vi "SATTPdll.vi"(8 "error in (no error)":errorcluster, 11 "SAT Inputs":T2={"t"=0.0, "p"=0.0, "z"=[0.0, 0.0, 0.0, 0.0, 0.0, 0.0, 0.0, 0.0, 0.0, 0.0, 0.0, 0.0, 0.0, 0.0, 0.0, 0.0, 0.0, 0.0, 0.0, 0.0], "kph"=0, "iGuess"=0} {"kph" items=["0 - Flash calculation (T and P known)", "1 - T and xliq known, P and xvap returned", "2 - T and xvap known, P and xliq returned", "3 - P and xliq known, T and xvap returned", "4 - P and xvap known, T and xliq returned"]}) -> (0 "error out":errorcluster, 3 "SAT Outputs":T1={"D"=nan, "e"=nan, "h"=nan, "p"=nan, "s"=nan, "t"=nan, "q"=nan, "Dl"=nan, "Dv"=nan, "x"=[nan, nan, 0.0, 0.0, 0.0, 0.0, 0.0, 0.0, 0.0, 0.0, 0.0, 0.0, 0.0, 0.0, 0.0, 0.0, 0.0, 0.0, 0.0, 0.0], "y"=[nan, nan, 0.0, 0.0, 0.0, 0.0, 0.0, 0.0, 0.0, 0.0, 0.0, 0.0, 0.0, 0.0, 0.0, 0.0, 0.0, 0.0, 0.0, 0.0], "nroot"=0, "k1"=0, "t1"=nan, "p1"=nan, "d1"=nan, "k2"=0, "t2"=nan, "p2"=nan, "d2"=nan, "k3"=0, "t3"=nan, "p3"=nan, "d3"=nan, "ierr"=0, "herr"="", "herr_length"=0})   [LabVIEW 2016]
doc: "subroutine SATTPdll(t, p, z, kph, iguess, d, dl, dv, x, y, q, ierr, herr, herr_length)\n\nCalculate saturation properties for bubble, dew, or 2-phase states with the use of analytical derivatives of the Helmholtz energy with respect to composition.\n\nINPUTS:\n t--temperature [K] (input or output)\n p--pressure [MPa] (input or output)\n z--composition [array of mol frac]\n kph--Phase flag: 0 - Flash calculation (T and P known)\n 1 - T and x known, P and y returned\n 2 - T and y known, P and x returned\n 3 - P and x known, T and y returned\n 4 - P and y known, T and x returned\n if this value is negative, the retrograde point will be returned\n iGuess--if set to 1, all inputs are used as initial guesses for the calculation\n\nOUTPUTS:\n D--overall molar density [mol/L]\n Dl--molar density [mol/L] of saturated liquid\n Dv--molar density [mol/L] of saturated vapor\n x--liquid phase composition [array of mol frac]\n y--vapor phase composition [array of mol frac]\n q--quality\n ierr--error flag: 0 = successful\n 1 = unsuccessful\n herr--error string (character*255 variable if ierr<>0)\n herr_length-- length of variable herr (default: 255)"
uses:
  Ctl/SAT_Outputs.ctl
  REFPROP.DLL
panel:
  # "REFPROP-SATTP_dll.vi"
  # "subroutine SATTPdll(t, p, z, kph, iguess, d, dl, dv, x, y, q, ierr, herr, herr_length)"
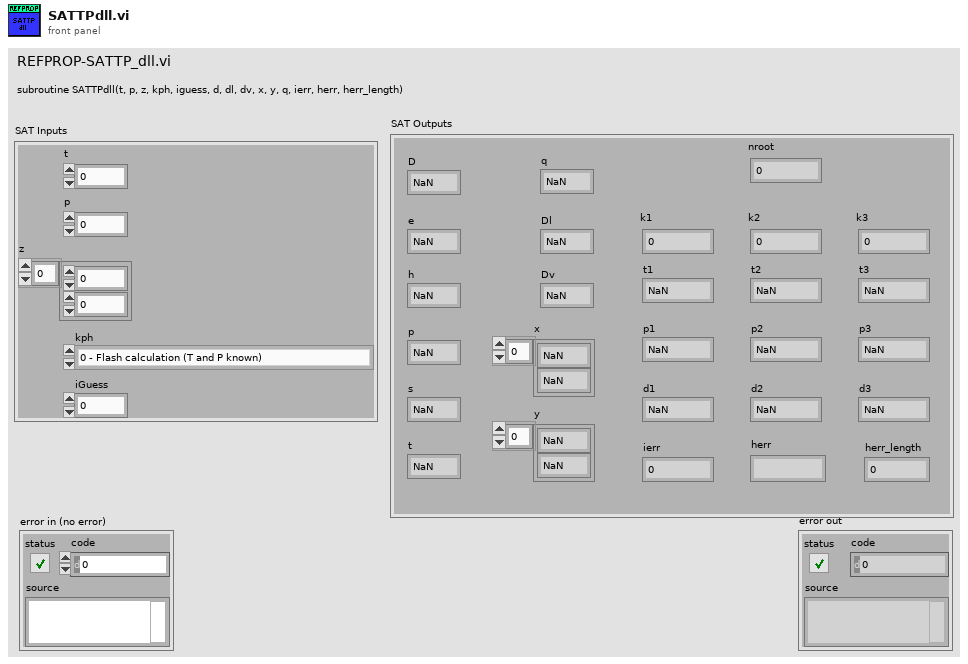
[diagram p1: front panel]
types:
  T1 = typedef "SAT_Outputs.ctl" = cluster{"D":dbl, "e":dbl, "h":dbl, "p":dbl, "s":dbl, "t":dbl, "q":dbl, "Dl":dbl, "Dv":dbl, "x":dbl[], "y":dbl[], "nroot":i32, "k1":i32, "t1":dbl, "p1":dbl, "d1":dbl, "k2":i32, "t2":dbl, "p2":dbl, "d2":dbl, "k3":i32, "t3":dbl, "p3":dbl, "d3":dbl, "ierr":i32, "herr":string, "herr_length":i32}
  T2 = cluster{"t":dbl, "p":dbl, "z":dbl[], "kph":u16, "iGuess":i32}
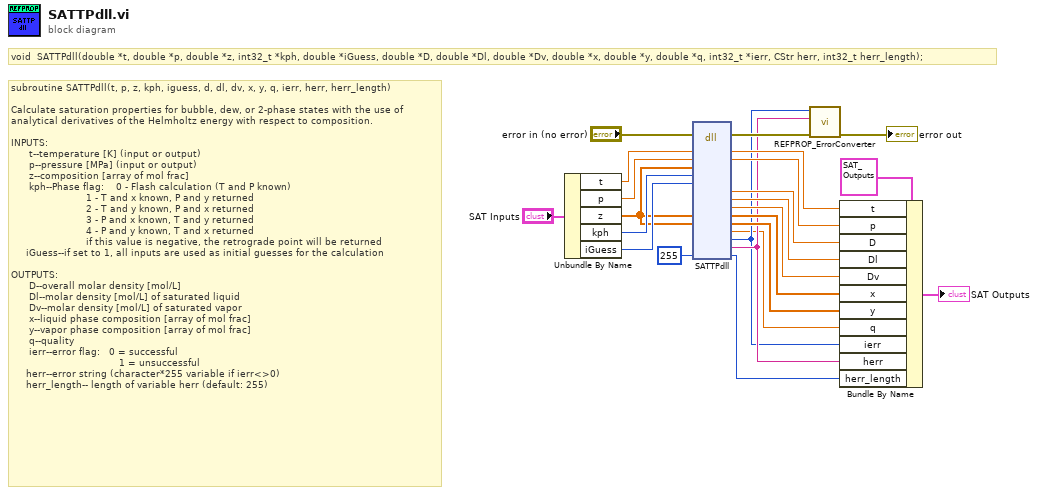
[diagram p0: block diagram]
diagram:
  # "void  SATTPdll(double *t, double *p, double *z, int32_t *kph, double *iGuess, double *D, double *Dl, double *Dv, double *x, double *y, double *q, int32_t *ierr, CStr herr, int32_t herr_length);"
  # "subroutine SATTPdll(t, p, z, kph, iguess, d, dl, dv, x, y, q, ierr, herr, herr_length)\n\nCalculate saturation properties for bubble, dew, or 2-phase states with the use of analytical derivatives of the Helmholtz energy with respect to composition.\n\nINPUTS:\n      t--temperature [K] (input or output)\n      p--pressure [MPa] (input or output)\n      z--composition [array of mol frac]\n      kph--Phase flag:    0 - Flash calculation (T and P known)\n                         1 - T and x known, P and y returned\n                         2 - T and y known, P and x returned\n                         3 - P and x known, T and y returned\n                         4 - P and y known, T and x returned\n                         if this value is negative, the retrograde point will be returned\n     iGuess--if set to 1, all inputs are used as initial guesses for the calculation\n\nOUTPUTS:\n      D--overall molar density [mol/L]\n      Dl--molar density [mol/L] of saturated liquid\n      Dv--molar density [mol/L] of saturated vapor\n      x--liquid phase composition [array of mol frac]\n      y--vapor phase composition [array of mol frac]\n      q--quality\n      ierr--error flag:   0 = successful\n                                    1 = unsuccessful\n     herr--error string (character*255 variable if ierr<>0)\n     herr_length-- length of variable herr (default: 255)"
  n1 = Unbundle By Name("SAT Inputs") -> ("t"=w21:dbl, "p"=w20:dbl, "z"=w14:dbl[], "kph"=w19:u16, "iGuess"=w18:i32)
  n2 = dll-call lib="C:/Program Files (x86)/REFPROP/REFPROP.*" fn="SATTPdll"(error in="error in (no error)", "t"=w21, "p"=w20, "z"=w14, "kph"=w19, "iGuess"=w18, "x"=w14, "y"=w14, "herr_length"=255 ("ln")) -> (error out=w22:errorcluster, "t"=w8:dbl, "p"=w7:dbl, "D"=w6:dbl, "Dl"=w12:dbl, "Dv"=w11:dbl, "x"=w10:dbl[], "y"=w9:dbl[], "q"=w1:dbl, "ierr"=w2:i32, "herr"=w3:string, "herr_length"=w4:i32)  [unwired: 12 in, 1 out]
  n3 = call "REFPROP_ErrorConverter.vi"("error in (no error)"=w22, "Error Message"=w3, "Error Code"=w2) -> ("error out"=→"error out":errorcluster)  [unwired: 8 in]
  n4 = Bundle By Name(cluster=T1 {"D"=nan, "e"=nan, "h"=nan, "p"=nan, "s"=nan, "t"=nan, "q"=0.0, "Dl"=nan, "Dv"=nan, "x"=[nan, nan, 0.0, 0.0, 0.0, 0.0, 0.0, 0.0, 0.0, 0.0, 0.0, 0.0, 0.0, 0.0, 0.0, 0.0, 0.0, 0.0, 0.0, 0.0], "y"=[nan, nan, 0.0, 0.0, 0.0, 0.0, 0.0, 0.0, 0.0, 0.0, 0.0, 0.0, 0.0, 0.0, 0.0, 0.0, 0.0, 0.0, 0.0, 0.0], "nroot"=0, "k1"=0, "t1"=nan, "p1"=nan, "d1"=nan, "k2"=0, "t2"=nan, "p2"=nan, "d2"=nan, "k3"=0, "t3"=nan, "p3"=nan, "d3"=nan, "ierr"=0, "herr"="", "herr_length"=0} ("SAT Outputs"), "t"=w8, "p"=w7, "D"=w6, "Dl"=w12, "Dv"=w11, "x"=w10, "y"=w9, "q"=w1, "ierr"=w2, "herr"=w3, "herr_length"=w4) -> (→"SAT Outputs":T1)
